vi "DataHandler Type.vi"(8 "error in (no error)":errorcluster, 11 "ScalingDataHandler in":refnum<class "ScalingDataHandler.lvclass">) -> (0 "error out":errorcluster, 2 "DataHandler Type":string, 3 "ScalingDataHandler out":refnum<class "ScalingDataHandler.lvclass">)   [LabVIEW 2020, in "VolatusDataProcessing.lvlib" / "ScalingDataHandler.lvclass"]
uses:
  ScalingDataHandler.lvclass
  ScalingDataHandler.lvclass/ScalingDataHandler.ctl
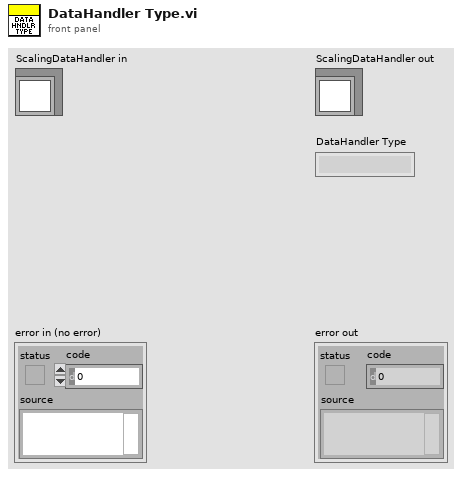
[diagram p1: front panel]
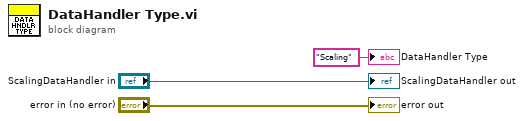
[diagram p0: block diagram]
diagram:
  "error out" <- "error in (no error)"
  "ScalingDataHandler out" <- "ScalingDataHandler in"
  "DataHandler Type" <- "Scaling" ("DataHandler Type")
